vi "Get Channel By Name.vi"(8 "error in":errorcluster, 10 "Channel Name":string, 11 "Item Ref in":refnum<data-value>) -> (0 "error out":errorcluster, 3 "Channel Ref out":refnum<data-value>)   [LabVIEW 2024, in "Config File Parser.lvlib" / "Channel.lvclass"]
uses:
  Channel.lvclass
  Channel.lvclass/Channel.ctl
  Item/Item.lvclass
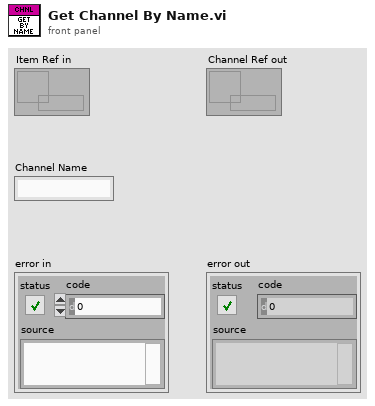
[diagram p1: front panel]
types:
  T1 = typedef "Config File Parser.lvlib/Item.lvclass/Item Type.ctl" = enum16{"Channel", "Section"}
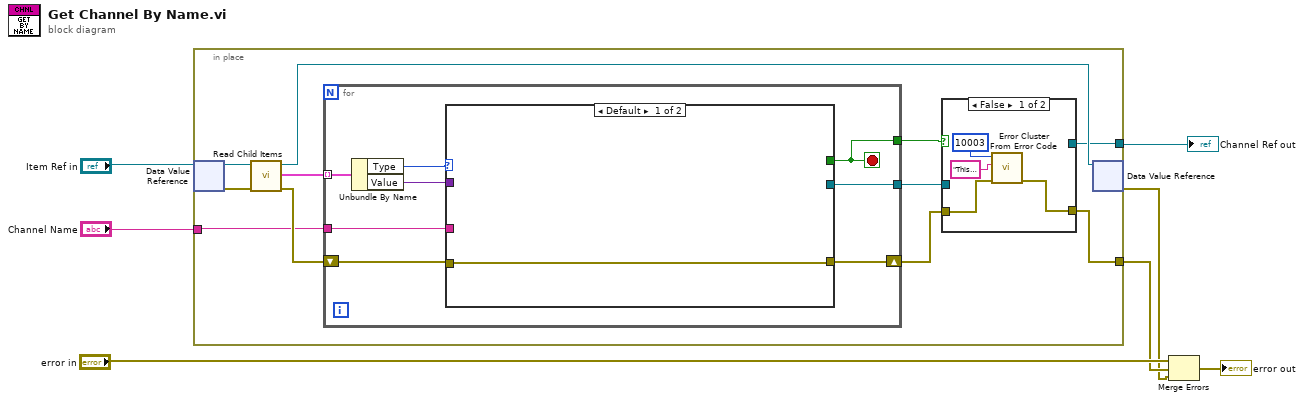
[diagram p0: block diagram]
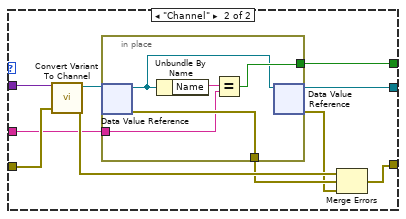
[diagram p3: hidden frame]
diagram:
  n1 = in-place "In Place Element Structure" {
    in-place-border: "Channel Name" -> [w12]
    in-place-border: [w15] -> w6
    in-place-border: [w8] -> w1
    n2 = in-place-dvr #1("Item Ref in") -> (w14:refnum<class "Item.lvclass">, w18:errorcluster)
    n3 = call-dynamic "Read Child Items.vi"("error in"=w18, "Item in"=w14) -> ("error out"=w17:errorcluster, "Child Items"=w13:cluster{"Type":T1, "Value":variant}[], "Item out"=w11:refnum<class "Item.lvclass">)  [unwired: 7 in]
    n4 = for {
      tunnel: w13 -> [w30] mode=indexing
      tunnel: w12 -> [w27]
      shift-right: [w31] -> w16
      shift-left: w17 -> [w32]
      tunnel: [w26] -> w10
      tunnel: [w25] -> w9
      stop <- w26 stop-if-true
      n5 = Unbundle By Name(w30) -> ("Type"=w29:T1, "Value"=w28:variant)
      n6 = case shown="Default" w29 {
        tunnel: w28 -> [_ w38]
        tunnel: w27 -> [_ w36]
        tunnel: [_ w35] -> w26
        tunnel: [_ w34] -> w25
        tunnel: w32 -> [w33 w43]
        tunnel: [w33 w39] -> w31
        frame Default {
        }
        frame "Channel" {
          n7 = call "Convert Variant To Channel.vi"("error in"=w43, "Channel Variant"=w38) -> ("error out"=w42:errorcluster, "Channel Ref out"=w37:refnum<data-value>)  [unwired: 8 in]
          n8 = in-place "In Place Element Structure" {
            in-place-border: w36 -> [w46]
            in-place-border: [w45] -> w35
            in-place-border: [w48] -> w41
            n9 = in-place-dvr #2(w37) -> (w44:refnum<class "Channel.lvclass">, w48:errorcluster)
            n10 = Unbundle By Name(w44) -> ("Name"=w47:string)
            n11 = Equal?(x=w47, y=w46) -> (x = y?=w45:bool)
            n12 = in-place-dvr #2(w44) -> (w34:refnum<data-value>, w40:errorcluster)
          }
          n13 = Merge Errors(w42, w41, w40) -> (w39:errorcluster)
        }
      }
    }
    n14 = case shown="False" w10 {
      tunnel: w16 -> [w22 w24]
      tunnel: [w21 w24] -> w15
      tunnel: w9 -> [_ w23]
      tunnel: [_ w23] -> w8
      frame False {
        n15 = call <vilib>:"Error Cluster From Error Code.vi"("error in (no error)"=w22, "error message (\"\")"="This Channel Does not exist.", "error code (0)"=10003) -> ("error out"=w21:errorcluster)  [unwired: 6 in]
      }
      frame True {
      }
    }
    n16 = in-place-dvr #1(w11) -> (w5:errorcluster)  [unwired: 1 out]
  }
  "Channel Ref out" <- w1
  n17 = Merge Errors("error in", w6, w5) -> (→"error out":errorcluster)
